vi "Save calibration profile.vi"(8 "error in (no error)":errorcluster, 9 "Col Headers":string[](array[string]), 10 "LB data full":string[][](array[string]), 11 "Image Sequence":T1[](array[typedef])) -> (0 "Error Out":errorcluster, 3 "created folder path":path)   [LabVIEW 2020]
uses:
  <vilib>/vision/Image Controls.llb/IMAQ Image.ctl
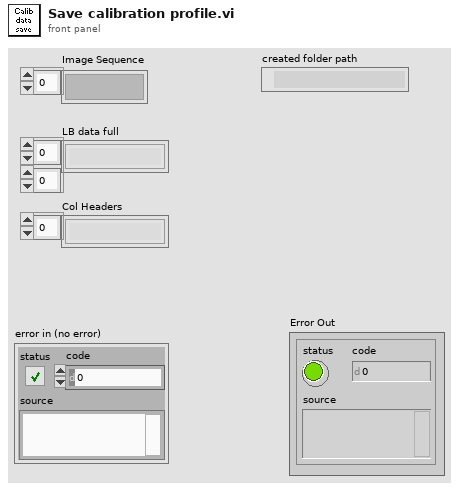
[diagram p1: front panel]
types:
  T1 = typedef "IMAQ Image.ctl" = refnum<image>
  T2 = enum16{"open", "replace", "create", "open or create", "replace or create", "replace or create with confirmation"}
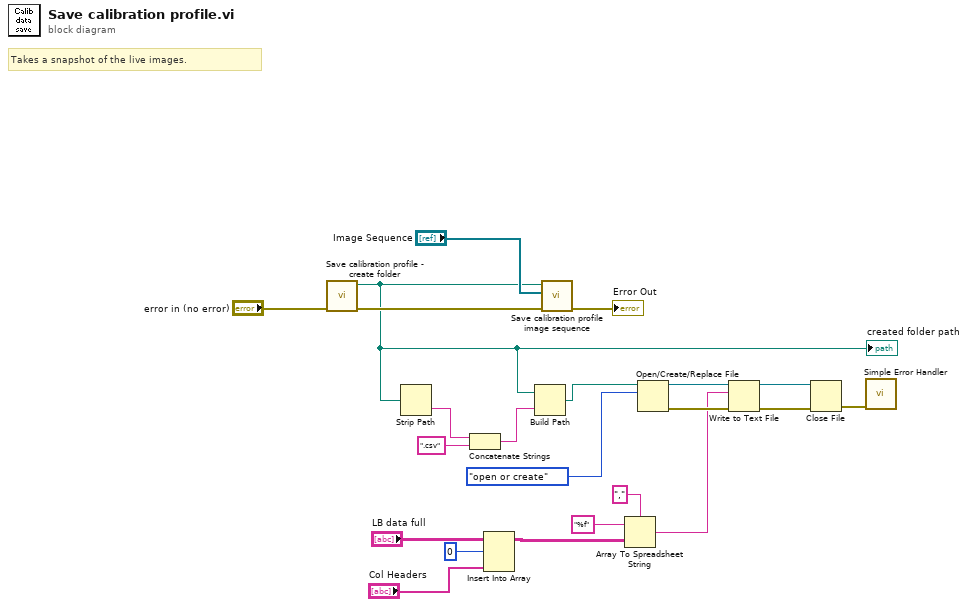
[diagram p0: block diagram]
diagram:
  # "Takes a snapshot of the live images."
  n1 = call "Save calibration profile - create folder.vi"("error in (no error)"="error in (no error)") -> ("error out"=w22:errorcluster, "created path"=w1:path)  [unwired: 8 in, 1 out]
  "created folder path" <- w1
  n2 = Strip Path(path=w1) -> (name=w2:string)  [unwired: 1 out]
  n3 = Concatenate Strings(w2, ".csv" ("string")) -> (w17:string)
  n4 = Insert Into Array(array="LB data full", index (row)=0, new element="Col Headers") -> (w9:string[][])  [unwired: 1 in]
  n5 = Build Path(base path=w1, name or relative path=w17) -> (appended path=w6:path)
  n6 = call "Save calibration profile image sequence.vi"("Error In"=w22, "Image In"="Image Sequence", "folder path"=w1) -> ("Error Out"=→"Error Out":errorcluster)  [unwired: 8 in]
  n7 = Array To Spreadsheet String(delimiter (Tab)=",", array=w9, 3:"%f" ("format string")) -> (spreadsheet string=w3:string)
  n8 = Open/Create/Replace File(file path (use dialog)=w6, operation (0:open)=T2."open or create") -> (refnum out=w16:refnum<file>, error out=w15:errorcluster)  [unwired: 4 in, 1 out]
  n9 = Write to Text File(file (use dialog)=w16, text=w3, error in=w15) -> (refnum out=w13:refnum<file>, error out=w14:errorcluster)  [unwired: 1 in, 1 out]
  n10 = Close File(refnum=w13, error in=w14) -> (error out=w4:errorcluster)  [unwired: 1 out]
  n11 = call <vilib>:"Simple Error Handler.vi"("error in (no error)"=w4) -> ()  [unwired: 4 in, 5 out]
